vi "error.vi"(1 "Boolean":bool, 2 "millisecond timer value":u32, 3 "reference":refnum<vi>, 4 "error message":refnum<vi>) -> (0 "millisecond timer value 2":u32)   [LabVIEW 2020]
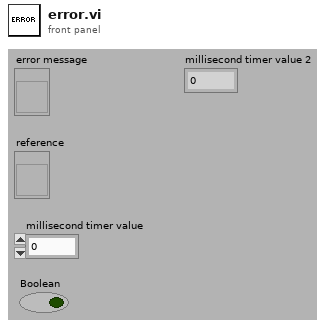
[diagram p1: front panel]
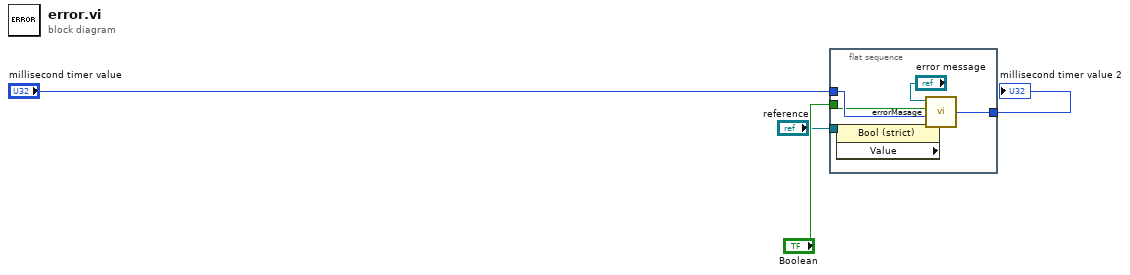
[diagram p0: block diagram]
diagram:
  n1 = flat-sequence {
    tunnel: [w10] -> w2
    tunnel: "millisecond timer value" -> [w9]
    tunnel: "Boolean" -> [w7]
    tunnel: "reference" -> [w5]
    frame #0 {
      n2 = property class="Bool (strict)"(reference=w5) -> ("Value"=w6:bool)  [unwired: 1 in, 2 out]
      n3 = call "errorMasage.vi"("error (h)"=w6, "millisecond timer value"=w9, "Boolean"=w7, "error message"="error message") -> ("millisecond timer value 2"=w10:u32)
    }
  }
  "millisecond timer value 2" <- w2
